vi "snap_calibration_images.vi"(8 "error in (no error)":errorcluster, 10 "Number of Frames to Get":u32, 11 "Session In":T1) -> (0 "error out":errorcluster, 3 "Image Out":T2)   [LabVIEW 2019]
uses:
  <vilib>/vision/Image Controls.llb/IMAQ Image.ctl
  <vilib>/userDefined/High Color/IMAQdx.ctl
  <vilib>/vision/driver/IMAQdx.llb/IMAQdx Buffer Number Mode.ctl
  <vilib>/vision/driver/NI_Vision_Acquisition_Software.lvlib
  <vilib>/vision/NI_Vision_Development_Module.lvlib
panel:
  out "CameraBuffer Number":u32
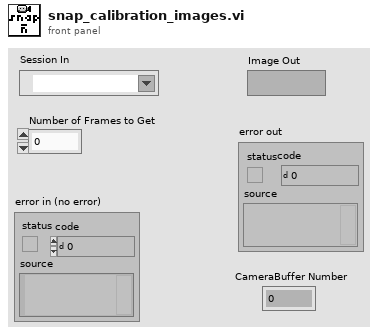
[diagram p1: front panel]
types:
  T1 = typedef "IMAQdx.ctl" = refnum<k21>
  T2 = typedef "IMAQ Image.ctl" = refnum<image>
  T3 = typedef "Image Type" = u32
  T4 = typedef "NI_Vision_Acquisition_Software.lvlib/IMAQdx Buffer Number Mode.ctl" = enum32{"Next", "Last", "Buffer Number", "Every", "Last New"}
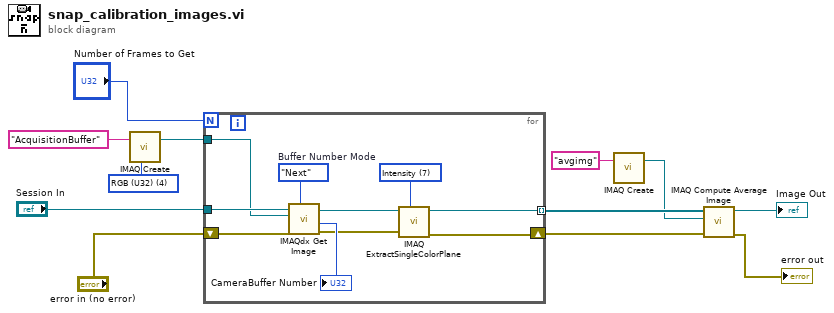
[diagram p0: block diagram]
diagram:
  w11 = T3 4 items=["Grayscale (U8)", "Grayscale (I16)", "Grayscale (SGL)", "Complex (CSG)", "RGB (U32)", "HSL (U32)", "RGB (U64)"] ("Image Type")
  n1 = call "IMAQ Create"("Image Name"="AcquisitionBuffer", "Image Type"=w11) -> ("New Image"=w10:T2)  [unwired: 3 in, 1 out]
  n2 = for {
    N: "Number of Frames to Get" -> [_]
    tunnel: w10 -> [w19]
    tunnel: "Session In" -> [w20]
    tunnel: [w15] -> w7 mode=indexing
    shift-right: [w13] -> w5
    shift-left: "error in (no error)" -> [w14]
    w18 = 7 items=["Red", "Green", "Blue", "Hue", "Saturation", "Luminance", "Value", "Intensity"] ("Color Plane")
    w22 = IMAQdx_Buffer_Number_Mode."Next"  # Buffer Number Mode
    n3 = call <vilib>:"IMAQdx Get Image.vi"("Buffer Number Mode (Next)"=w22, "error in"=w14, "Image In"=w19, "Session In"=w20) -> ("error out"=w16:errorcluster, "Buffer Number Out"=→"CameraBuffer Number":u32, "Image Out"=w17:T2)  [unwired: 4 in, 1 out]
    n4 = call "IMAQ ExtractSingleColorPlane"("Color Plane"=w18, "error in (no error)"=w16, "Image Src"=w17) -> ("error out"=w13:errorcluster, "Image Dst Out"=w15:T2)  [unwired: 7 in]
  }
  n5 = call "IMAQ Create"("Image Name"="avgimg") -> ("New Image"=w2:T2)  [unwired: 4 in, 1 out]
  n6 = call "IMAQ Compute Average Image"("error in (no error)"=w5, "Image Dst"=w2, "Images"=w7) -> ("error out"=→"error out":errorcluster, "Image Dst Out"=→"Image Out":T2)  [unwired: 7 in]
